vi "Calculate pO2-Rev3.vi"(10 "Spectral Data":T4={"PDT Amp [v]"=0.0, "RIS Amp [v]"=0.0, "B-Field"=[], "All In-Phase Scan Spectra"=[], "Model Select"=enum."OneCompRISTwoPDT", "Fit Each Scan"=FALSE, "PDT Center [g]"=0.0, "In-Phase Average Spectra"=[], "In-Phase Median Spectra"=[], "Out-Phase Median Spectra"=[], "Out-Phase Average Spectra"=[], "Fit Spectra"=[], "Fit No-Baseline Spectra"=[], "All Out-Phase Scan Spectra"=[], "Baseline Offset Correction"=FALSE, "In-Phase Offset [v]"=0.0, "Out-Phase Offset [v]"=0.0, "Ch2 Input\n(Balance)"=[], "Ch3 Input\n(Phase)"=[], "Ch4 Input\n(AFC)"=[], "Fit Pars"=[], "Fit Pars Errors"=[], "Fit Pars Labels"=[], "Raw Scan DAQ Data"=[], "Bad Scans Indicies"=[], "Good In-Phase Scan Spectra"=[], "Good Out-Phase Scan Spectra"=[], "Bad In-Phase Scan Spectra"=[], "Bad Out-Phase Scan Spectra"=[], "Number of bad scans"=0, "Fit History"=[], "PDT Amp. History/Set [v]"=[], "RIS Amp. History/Set [v]"=[], "RIS Amp. History/Scan [v]"=[], "All Shifted B-Fields"=[], "Good Shifted B-Fields"=[], "Ch5 Input\n(SpO2)"=[], "Ch6 Input\n(BPM)"=[], "Global SNR"=0.0, "Fit Error History"=[], "SNR History"=[]} {"Global SNR" min=0.0; "PDT Center [g]" min=0.0; "RIS Amp [v]" min=0.0; "PDT Amp [v]" min=0.0}, 11 "Measurement Information":T1={"Comments"="", "Directory Input"="", "Data file path"=path "C:/Data/EPR Data", "Scripting File"=path "C:/Data/Configuration Script.csv", "Save Data"=FALSE, "Tooth size (d11) [mm]"=0.0, "Tooth size (d12) [mm]"=0.0, "Tooth size (d21) [mm]"=0.0, "Tooth size (d22) [mm]"=0.0, "Dose of Tooth [Gy]"=0.0, "Safe Shutdown?"=FALSE, "Gases Available"=[], "Database Username"="", "Database Password"="", "Database Login URL"="", "Database Upload URL"="", "Database Success URL"="", "Database XML URL"="", "Database Resonator URL"="", "Session Number"=0, "Set #"=0, "Resonator Operator"="", "Session Type"="", "Tooth/Sample ID"="", "Volunteer ID"="", "Computer Operator"="", "Volunteer Type"="", "Site/Tooth Selection (T8,T9)"="", "Resonator"="", "Measurement Site"="", "Non-standard session?"=FALSE, "EPR DAQ Version"="", "Session Path"=path "C:/Data/EPR Data", "Chosen Applied State"="", "Chosen Initial State"="", "Time of Transition"="", "DAQ Mode"=enum."Engineering", "pO2/Scan [mmHg]"=[], "pO2/Set [mmHg]"=[], "Linewidth (HWHM)/Scan [Gauss]"=[], "Linewidth (HWHM)/Set [Gauss]"=[], "pO2 Conversion"="", "Dose Calibration Cluster"={"Dose Response"={"grand_mean"=0.0292016, "slope"=0.0188720543}, "Dose Correction"={"Sex"=1, "a0"=7.719669421, "a1"=-2.746550736, "a2"=-0.186490355, "a3"=0.041922063, "a4"=-0.849147359, "a5"=0.14330063, "a6"=0.019930219, "A_n"=40.0, "H_n"=10.12, "Dose Correction"=FALSE}, "Dose Reporting"={"Reporting is"=TRUE, "sd_threshold [AU]"=0.06, "sd_model [Gy]"=0.66, "dosimetric_threshold [Gy]"=2.0, "Add intrasession errors is"=FALSE, "Prior Radiation?"=FALSE}}, "OxyChip Slope"=0.0, "OxyChip Intercept"=0.0, "QA Mode"=enum."Select QA Mode", "QA Session?"=FALSE, "Sample Type"=enum."Empty Resonator", "Report pO2/Scan"=FALSE, "Skip End Session Save"=FALSE, "Number of sites"=enum."# Probes", "Recipient Name"="", "Sender Name"="", "Recipient Email"="", "Transition State History"=[], "pO2 Report Times"=[], "Temperature [C]"=0.0, "+Error pO2/Scan [mmHg]"=[], "-Error pO2/Scan [mmHg]"=[], "+Error pO2/Set [mmHg]"=[], "-Error pO2/Set [mmHg]"=[], "Oxy Phase Exclusion Tolerance [rad]"=0.0, "Oxy Center Exclusion Tolerance [%]"=0.0, "Oxy Exclude Unacceptable"=FALSE, "Oxy Unacceptable Estimate Flags"=[], "Save Session PPT"=FALSE, "Flagged Bad Sets"=[]} {"Oxy Center Exclusion Tolerance [%]" format="%#_9g"; "Oxy Phase Exclusion Tolerance [rad]" format="%#_9g"; "Temperature [C]" format="%#_9g"; "OxyChip Intercept" format="%#_9g"; "OxyChip Slope" format="%#_9g"; "Dose Calibration Cluster"."Dose Reporting"."dosimetric_threshold [Gy]" format="%#_9g"; "Dose Calibration Cluster"."Dose Reporting"."sd_model [Gy]" format="%#_9g"; "Dose Calibration Cluster"."Dose Reporting"."sd_threshold [AU]" format="%#_9g"; "Dose Calibration Cluster"."Dose Correction"."H_n" format="%#_9g"; "Dose Calibration Cluster"."Dose Correction"."A_n" format="%#_9g"; "Dose Calibration Cluster"."Dose Correction"."a6" format="%#.9g"; "Dose Calibration Cluster"."Dose Correction"."a5" format="%#.9g"; "Dose Calibration Cluster"."Dose Correction"."a4" format="%#.9g"; "Dose Calibration Cluster"."Dose Correction"."a3" format="%#.9g"; "Dose Calibration Cluster"."Dose Correction"."a2" format="%#.9g"; "Dose Calibration Cluster"."Dose Correction"."a1" format="%#.9g"; "Dose Calibration Cluster"."Dose Correction"."a0" format="%#.9g"; "Dose Calibration Cluster"."Dose Correction"."Sex" items=["Male"=1, "Female"=0]; "Dose Calibration Cluster"."Dose Response"."slope" format="%#_9g"; "Dose Calibration Cluster"."Dose Response"."grand_mean" format="%#_9g"}) -> (0 "pO2 Conversion":string, 1 "pO2 [mmHg]":dbl[](array[numeric]), 3 "Measurement Information Out":T1={"Comments"="", "Directory Input"="", "Data file path"=path "C:/Data/EPR Data", "Scripting File"=path "C:/Data/Configuration Script.csv", "Save Data"=FALSE, "Tooth size (d11) [mm]"=0.0, "Tooth size (d12) [mm]"=0.0, "Tooth size (d21) [mm]"=0.0, "Tooth size (d22) [mm]"=0.0, "Dose of Tooth [Gy]"=0.0, "Safe Shutdown?"=FALSE, "Gases Available"=[], "Database Username"="", "Database Password"="", "Database Login URL"="", "Database Upload URL"="", "Database Success URL"="", "Database XML URL"="", "Database Resonator URL"="", "Session Number"=0, "Set #"=0, "Resonator Operator"="", "Session Type"="", "Tooth/Sample ID"="", "Volunteer ID"="", "Computer Operator"="", "Volunteer Type"="", "Site/Tooth Selection (T8,T9)"="", "Resonator"="", "Measurement Site"="", "Non-standard session?"=FALSE, "EPR DAQ Version"="", "Session Path"=path "C:/Data/EPR Data", "Chosen Applied State"="", "Chosen Initial State"="", "Time of Transition"="", "DAQ Mode"=enum."Engineering", "pO2/Scan [mmHg]"=[], "pO2/Set [mmHg]"=[], "Linewidth (HWHM)/Scan [Gauss]"=[], "Linewidth (HWHM)/Set [Gauss]"=[], "pO2 Conversion"="", "Dose Calibration Cluster"={"Dose Response"={"grand_mean"=0.0292016, "slope"=0.0188720543}, "Dose Correction"={"Sex"=1, "a0"=7.719669421, "a1"=-2.746550736, "a2"=-0.186490355, "a3"=0.041922063, "a4"=-0.849147359, "a5"=0.14330063, "a6"=0.019930219, "A_n"=40.0, "H_n"=10.12, "Dose Correction"=FALSE}, "Dose Reporting"={"Reporting is"=TRUE, "sd_threshold [AU]"=0.06, "sd_model [Gy]"=0.66, "dosimetric_threshold [Gy]"=2.0, "Add intrasession errors is"=FALSE, "Prior Radiation?"=FALSE}}, "OxyChip Slope"=0.0, "OxyChip Intercept"=0.0, "QA Mode"=enum."Select QA Mode", "QA Session?"=FALSE, "Sample Type"=enum."Empty Resonator", "Report pO2/Scan"=FALSE, "Skip End Session Save"=FALSE, "Number of sites"=enum."# Probes", "Recipient Name"="", "Sender Name"="", "Recipient Email"="", "Transition State History"=[], "pO2 Report Times"=[], "Temperature [C]"=0.0, "+Error pO2/Scan [mmHg]"=[], "-Error pO2/Scan [mmHg]"=[], "+Error pO2/Set [mmHg]"=[], "-Error pO2/Set [mmHg]"=[], "Oxy Phase Exclusion Tolerance [rad]"=0.0, "Oxy Center Exclusion Tolerance [%]"=0.0, "Oxy Exclude Unacceptable"=FALSE, "Oxy Unacceptable Estimate Flags"=[], "Save Session PPT"=FALSE, "Flagged Bad Sets"=[]} {"Oxy Center Exclusion Tolerance [%]" format="%#_9g"; "Oxy Phase Exclusion Tolerance [rad]" format="%#_9g"; "Temperature [C]" format="%#_9g"; "OxyChip Intercept" format="%#_9g"; "OxyChip Slope" format="%#_9g"; "Dose Calibration Cluster"."Dose Reporting"."dosimetric_threshold [Gy]" format="%#_9g"; "Dose Calibration Cluster"."Dose Reporting"."sd_model [Gy]" format="%#_9g"; "Dose Calibration Cluster"."Dose Reporting"."sd_threshold [AU]" format="%#_9g"; "Dose Calibration Cluster"."Dose Correction"."H_n" format="%#_9g"; "Dose Calibration Cluster"."Dose Correction"."A_n" format="%#_9g"; "Dose Calibration Cluster"."Dose Correction"."a6" format="%#.9g"; "Dose Calibration Cluster"."Dose Correction"."a5" format="%#.9g"; "Dose Calibration Cluster"."Dose Correction"."a4" format="%#.9g"; "Dose Calibration Cluster"."Dose Correction"."a3" format="%#.9g"; "Dose Calibration Cluster"."Dose Correction"."a2" format="%#.9g"; "Dose Calibration Cluster"."Dose Correction"."a1" format="%#.9g"; "Dose Calibration Cluster"."Dose Correction"."a0" format="%#.9g"; "Dose Calibration Cluster"."Dose Correction"."Sex" items=["Male"=1, "Female"=0]; "Dose Calibration Cluster"."Dose Response"."slope" format="%#_9g"; "Dose Calibration Cluster"."Dose Response"."grand_mean" format="%#_9g"}, 4 "Negative pO2 Error [mmHg]":dbl[](array[numeric]), 6 "Positive pO2 Error [mmHg]":dbl[](array[numeric]))   [LabVIEW 2016]
uses:
  Types/Measurement Information.ctl
  Dose Calculation and Reporting/Dose Calculation Control.ctl
  Types/Sample Type.ctl
  Types/Spectral Data.ctl
  Types/Fitting Model Selection.ctl
panel:
  # "Session Information"
  # "Oximetric Data and Information"
  # "Email"
  # "Tooth Information"
  # "Database"
  # "Session Information"
  # "Oximetric Data and Information"
  # "Email"
  # "Tooth Information"
  # "Database"
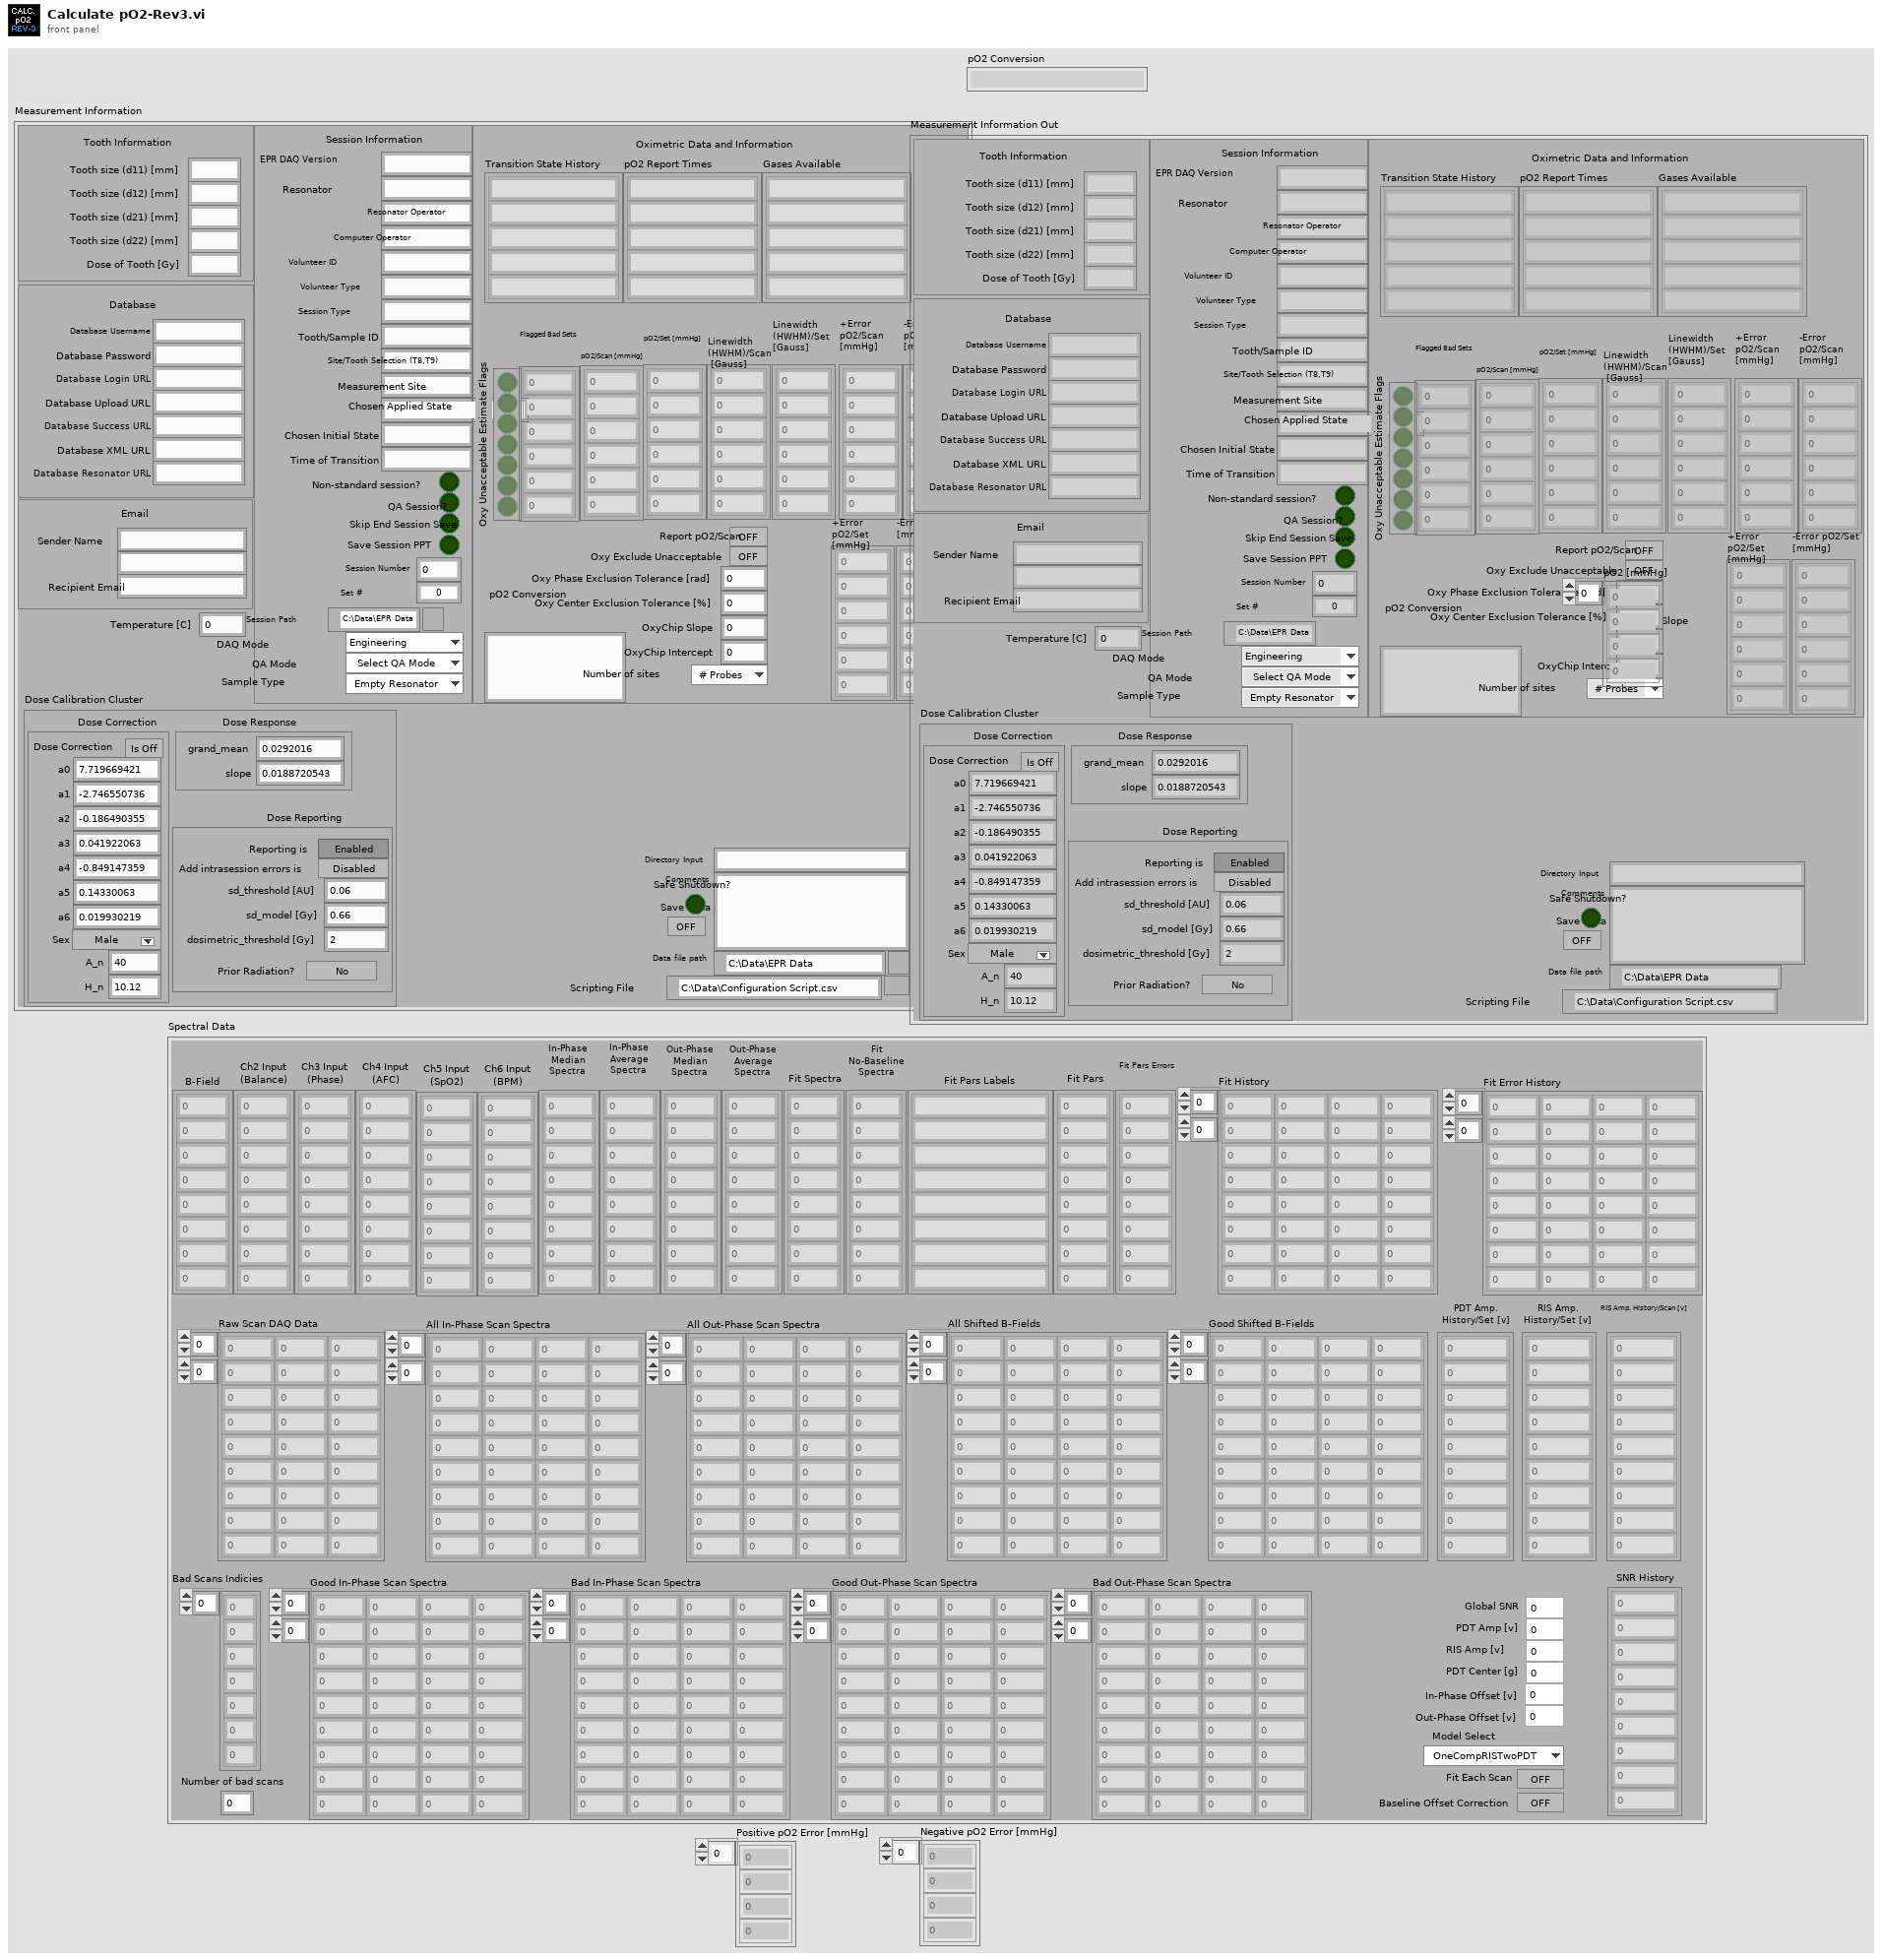
[diagram p1: front panel]
types:
  T1 = typedef "Measurement Information.ctl" = cluster{"Comments":string, "Directory Input":string, "Data file path":path, "Scripting File":path, "Save Data":bool, "Tooth size (d11) [mm]":dbl, "Tooth size (d12) [mm]":dbl, "Tooth size (d21) [mm]":dbl, "Tooth size (d22) [mm]":dbl, "Dose of Tooth [Gy]":dbl, "Safe Shutdown?":bool, "Gases Available":string[], "Database Username":string, "Database Password":string, "Database Login URL":string, "Database Upload URL":string, "Database Success URL":string, "Database XML URL":string, "Database Resonator URL":string, "Session Number":i32, "Set #":u32, "Resonator Operator":string, "Session Type":string, "Tooth/Sample ID":string, "Volunteer ID":string, "Computer Operator":string, "Volunteer Type":string, "Site/Tooth Selection (T8,T9)":string, "Resonator":string, "Measurement Site":string, "Non-standard session?":bool, "EPR DAQ Version":string, "Session Path":path, "Chosen Applied State":string, "Chosen Initial State":string, "Time of Transition":string, "DAQ Mode":enum16{"Engineering", "Dosimetry", "Oximetry"}, "pO2/Scan [mmHg]":dbl[][], "pO2/Set [mmHg]":dbl[][], "Linewidth (HWHM)/Scan [Gauss]":dbl[][], "Linewidth (HWHM)/Set [Gauss]":dbl[][], "pO2 Conversion":string, "Dose Calibration Cluster":T2, "OxyChip Slope":dbl, "OxyChip Intercept":dbl, "QA Mode":enum16{"Select QA Mode", "QA-Start/End", "QA-Mid", "QA-Weekly", "QA-Eng", "Check Calibration"}, "QA Session?":bool, "Sample Type":T3, "Report pO2/Scan":bool, "Skip End Session Save":bool, "Number of sites":enum16{"# Probes", "1", "2", "3", "4"}, "Recipient Name":string, "Sender Name":string, "Recipient Email":string, "Transition State History":string[], "pO2 Report Times":string[], "Temperature [C]":dbl, "+Error pO2/Scan [mmHg]":dbl[][], "-Error pO2/Scan [mmHg]":dbl[][], "+Error pO2/Set [mmHg]":dbl[][], "-Error pO2/Set [mmHg]":dbl[][], "Oxy Phase Exclusion Tolerance [rad]":dbl, "Oxy Center Exclusion Tolerance [%]":dbl, "Oxy Exclude Unacceptable":bool, "Oxy Unacceptable Estimate Flags":bool[], "Save Session PPT":bool, "Flagged Bad Sets":u32[]}
  T2 = typedef "Dose Calculation Control.ctl" = cluster{"Dose Response":cluster{"grand_mean":dbl, "slope":dbl}, "Dose Correction":cluster{"Sex":u16, "a0":dbl, "a1":dbl, "a2":dbl, "a3":dbl, "a4":dbl, "a5":dbl, "a6":dbl, "A_n":dbl, "H_n":dbl, "Dose Correction":bool}, "Dose Reporting":cluster{"Reporting is":bool, "sd_threshold [AU]":dbl, "sd_model [Gy]":dbl, "dosimetric_threshold [Gy]":dbl, "Add intrasession errors is":bool, "Prior Radiation?":bool}}
  T3 = typedef "Sample Type.ctl" = enum16{"Empty Resonator", "IRS", "BallZero", "Irradiated Tooth", "Non-irradiated Tooth", "OxyChip", "LiPc", "PDT", "India Ink"}
  T4 = typedef "Spectral Data.ctl" = cluster{"PDT Amp [v]":dbl, "RIS Amp [v]":dbl, "B-Field":dbl[], "All In-Phase Scan Spectra":dbl[][], "Model Select":T5, "Fit Each Scan":bool, "PDT Center [g]":dbl, "In-Phase Average Spectra":dbl[], "In-Phase Median Spectra":dbl[], "Out-Phase Median Spectra":dbl[], "Out-Phase Average Spectra":dbl[], "Fit Spectra":dbl[], "Fit No-Baseline Spectra":dbl[], "All Out-Phase Scan Spectra":dbl[][], "Baseline Offset Correction":bool, "In-Phase Offset [v]":dbl, "Out-Phase Offset [v]":dbl, "Ch2 Input\n(Balance)":dbl[], "Ch3 Input\n(Phase)":dbl[], "Ch4 Input\n(AFC)":dbl[], "Fit Pars":dbl[], "Fit Pars Errors":dbl[], "Fit Pars Labels":string[], "Raw Scan DAQ Data":dbl[][], "Bad Scans Indicies":i32[], "Good In-Phase Scan Spectra":dbl[][], "Good Out-Phase Scan Spectra":dbl[][], "Bad In-Phase Scan Spectra":dbl[][], "Bad Out-Phase Scan Spectra":dbl[][], "Number of bad scans":i32, "Fit History":dbl[][], "PDT Amp. History/Set [v]":dbl[], "RIS Amp. History/Set [v]":dbl[], "RIS Amp. History/Scan [v]":dbl[], "All Shifted B-Fields":dbl[][], "Good Shifted B-Fields":dbl[][], "Ch5 Input\n(SpO2)":dbl[], "Ch6 Input\n(BPM)":dbl[], "Global SNR":dbl, "Fit Error History":dbl[][], "SNR History":dbl[]}
  T5 = typedef "Fitting Model Selection.ctl" = enum16{"OneCompRIS", "OneCompRISTwoPDT", "OneCompRISRev", "OneCompRISTwoPDTRev", "LiPc", "TwoLiPc", "ThreeLiPc", "FourLiPc", "PDTCalibration", "CE_Ink", "Printex", "MelaninTwoPDT"}
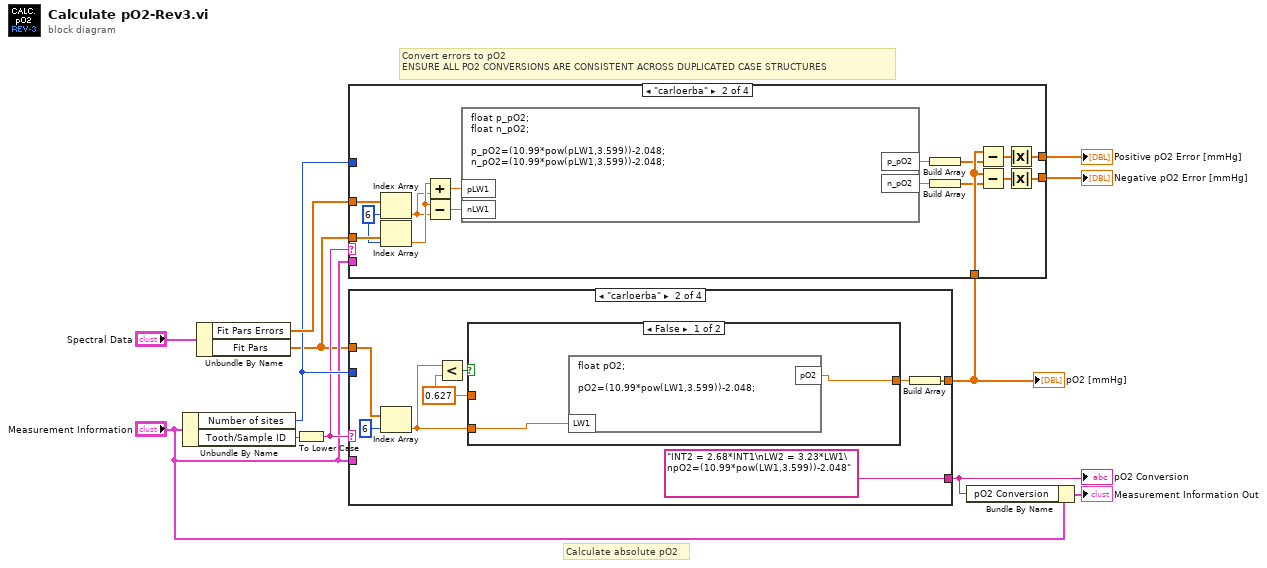
[diagram p0: block diagram]
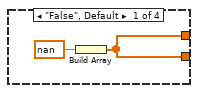
[diagram p2: hidden frame]
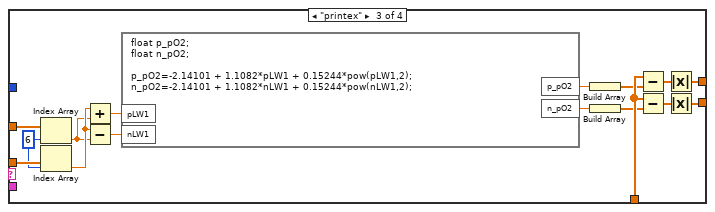
[diagram p3: hidden frame]
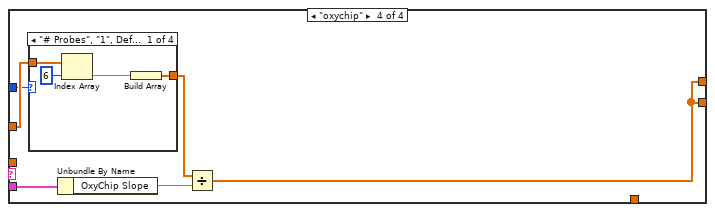
[diagram p4: hidden frame]
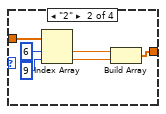
[diagram p5: hidden frame]
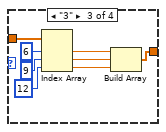
[diagram p6: hidden frame]
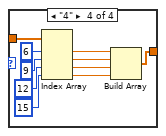
[diagram p7: hidden frame]
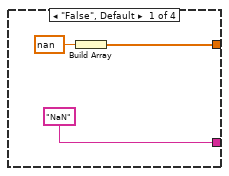
[diagram p8: hidden frame]
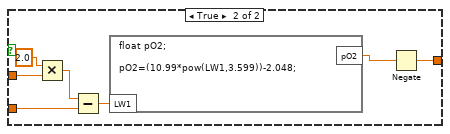
[diagram p9: hidden frame]
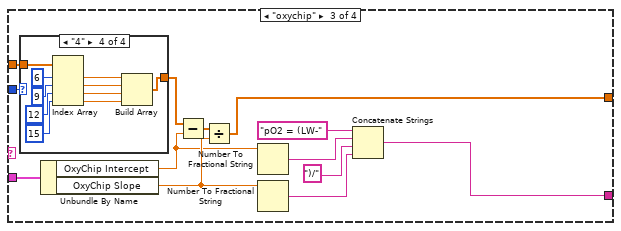
[diagram p10: hidden frame]
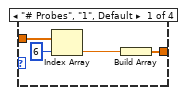
[diagram p11: hidden frame]
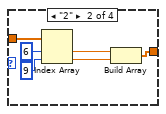
[diagram p12: hidden frame]
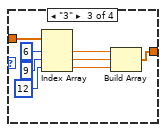
[diagram p13: hidden frame]
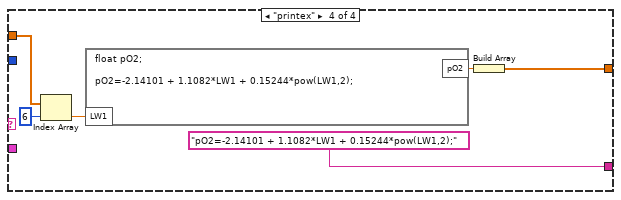
[diagram p14: hidden frame]
diagram:
  # "Calculate absolute pO2"
  # "Convert errors to pO2\nENSURE ALL PO2 CONVERSIONS ARE CONSISTENT ACROSS DUPLICATED CASE STRUCTURES"
  n1 = Unbundle By Name("Measurement Information") -> ("Number of sites"=w7:enum16{"# Probes", "1", "2", "3", "4"}, "Tooth/Sample ID"=w12:string)
  n2 = Unbundle By Name("Spectral Data") -> ("Fit Pars Errors"=w8:dbl[], "Fit Pars"=w4:dbl[])
  n3 = To Lower Case(string=w12) -> (all lower case string=w6:string)
  n4 = case shown="\"carloerba\"" w6 {
    tunnel: [w13 w20 w43 w74] -> w3
    tunnel: w4 -> [_ w22 w39 w76]
    tunnel: ["NaN" ("all lower case string") "INT2 = 2.68*INT1\nLW2 = 3.23*LW1\npO2=(10.99*pow(LW1,3.599))-2.048" ("all lower case string") w40 "pO2=-2.14101 + 1.1082*LW1 + 0.15244*pow(LW1,2);" ("all lower case string")] -> w10
    tunnel: "Measurement Information" -> [_ _ w45 _]
    tunnel: w7 -> [_ _ w37 _]
    frame "False", Default {
      n5 = Build Array(nan) -> (w13:dbl[])
    }
    frame "carloerba" {
      w16 = 0.627 ("y")
      n6 = Index Array(array=w22, index=6) -> (element=w17:dbl)
      n7 = Less?(x=w17, y=w16) -> (x < y?=w18:bool)
      n8 = case shown="False" w18 {
        tunnel: w17 -> [w25 w29]
        tunnel: [w24 w26] -> w19
        tunnel: w16 -> [_ w32]
        frame False {
          n9 = formula code="float pO2;\n\npO2=(10.99*pow(LW1,3.599))-2.048;"("LW1"=w25) -> ("pO2"=w24:dbl)
        }
        frame True {
          n10 = Multiply(x=2.0, y=w32) -> (x*y=w30:dbl)
          n11 = Subtract(x=w30, y=w29) -> (x-y=w28:dbl)
          n12 = formula code="float pO2;\n\npO2=(10.99*pow(LW1,3.599))-2.048;"("LW1"=w28) -> ("pO2"=w27:dbl)
          n13 = Negate(x=w27) -> (-x=w26:dbl)
        }
      }
      n14 = Build Array(w19) -> (w20:dbl[])
    }
    frame "oxychip" {
      n15 = case shown="\"4\"" w37 {
        tunnel: [w48 w54 w62 w72] -> w38
        tunnel: w39 -> [w46 w52 w60 w70]
        frame "# Probes", "1", Default {
          n16 = Index Array(array=w46, index=6) -> (element=w47:dbl)
          n17 = Build Array(w47) -> (w48:dbl[])
        }
        frame "2" {
          n18 = Index Array(array=w52, index #1=6 ("index"), index #2=9 ("index")) -> (element #1=w53:dbl, element #2=w50:dbl)
          n19 = Build Array(w53, w50) -> (w54:dbl[])
        }
        frame "3" {
          n20 = Index Array(array=w60, index #1=6 ("index"), index #2=9 ("index"), index #3=12 ("index")) -> (element #1=w61:dbl, element #2=w58:dbl, element #3=w56:dbl)
          n21 = Build Array(w61, w58, w56) -> (w62:dbl[])
        }
        frame "4" {
          n22 = Index Array(array=w70, index #1=6 ("index"), index #2=9 ("index"), index #3=12 ("index"), index #4=15 ("index")) -> (element #1=w71:dbl, element #2=w68:dbl, element #3=w66:dbl, element #4=w64:dbl)
          n23 = Build Array(w71, w68, w66, w64) -> (w72:dbl[])
        }
      }
      n24 = Unbundle By Name(w45) -> ("OxyChip Intercept"=w35:dbl, "OxyChip Slope"=w36:dbl)
      n25 = Subtract(x=w38, y=w35) -> (x-y=w44:dbl[])
      n26 = Divide(x=w44, y=w36) -> (x/y=w43:dbl[])
      n27 = Number To Fractional String(number=w35) -> (F-format string=w34:string)  [unwired: 3 in]
      n28 = Number To Fractional String(number=w36) -> (F-format string=w33:string)  [unwired: 3 in]
      n29 = Concatenate Strings("pO2 = (LW-" ("string"), w34, ")/" ("string"), w33) -> (w40:string)
    }
    frame "printex" {
      n30 = Index Array(array=w76, index=6) -> (element=w78:dbl)
      n31 = formula code="float pO2;\n\npO2=-2.14101 + 1.1082*LW1 + 0.15244*pow(LW1,2);"("LW1"=w78) -> ("pO2"=w77:dbl)
      n32 = Build Array(w77) -> (w74:dbl[])
    }
  }
  "pO2 Conversion" <- w10
  "pO2 [mmHg]" <- w3
  n33 = case shown="\"carloerba\"" w6 {
    tunnel: [w80 w82 w99 w114] -> w2
    tunnel: w8 -> [_ w97 w113 w118]
    tunnel: "Measurement Information" -> [_ _ _ w119]
    tunnel: w7 -> [_ _ _ w117]
    tunnel: [w80 w83 w98 w114] -> w1
    tunnel: w4 -> [_ w95 w111 _]
    tunnel: w3 -> [_ w86 w102 _]
    frame "False", Default {
      n34 = Build Array(nan) -> (w80:dbl[])
    }
    frame "carloerba" {
      w94 = 6 ("index")
      n35 = Index Array(array=w97, index=w94) -> (element=w89:dbl)
      n36 = Index Array(array=w95, index=w94) -> (element=w90:dbl)
      n37 = Add(x=w90, y=w89) -> (x+y=w93:dbl)
      n38 = Subtract(x=w90, y=w89) -> (x-y=w92:dbl)
      n39 = formula code="float p_pO2;\nfloat n_pO2;\n\np_pO2=(10.99*pow(pLW1,3.599))-2.048;\nn_pO2=(10.99*pow(pLW1,3.599))-2.048;"("pLW1"=w93, "nLW1"=w92) -> ("p_pO2"=w96:dbl, "n_pO2"=w91:dbl)
      n40 = Build Array(w96) -> (w85:dbl[])
      n41 = Build Array(w91) -> (w84:dbl[])
      n42 = Subtract(x=w86, y=w85) -> (x-y=w87:dbl[])
      n43 = Subtract(x=w86, y=w84) -> (x-y=w88:dbl[])
      n44 = Absolute Value(x=w87) -> (abs(x)=w82:dbl[])
      n45 = Absolute Value(x=w88) -> (abs(x)=w83:dbl[])
    }
    frame "printex" {
      w110 = 6 ("index")
      n46 = Index Array(array=w113, index=w110) -> (element=w105:dbl)
      n47 = Index Array(array=w111, index=w110) -> (element=w106:dbl)
      n48 = Add(x=w106, y=w105) -> (x+y=w109:dbl)
      n49 = Subtract(x=w106, y=w105) -> (x-y=w108:dbl)
      n50 = formula code="float p_pO2;\nfloat n_pO2;\n\np_pO2=-2.14101 + 1.1082*pLW1 + 0.15244*pow(pLW1,2);\nn_pO2=-2.14101 + 1.1082*nLW1 + 0.15244*pow(nLW1,2);"("pLW1"=w109, "nLW1"=w108) -> ("p_pO2"=w112:dbl, "n_pO2"=w107:dbl)
      n51 = Build Array(w112) -> (w100:dbl[])
      n52 = Build Array(w107) -> (w101:dbl[])
      n53 = Subtract(x=w102, y=w100) -> (x-y=w103:dbl[])
      n54 = Subtract(x=w102, y=w101) -> (x-y=w104:dbl[])
      n55 = Absolute Value(x=w103) -> (abs(x)=w99:dbl[])
      n56 = Absolute Value(x=w104) -> (abs(x)=w98:dbl[])
    }
    frame "oxychip" {
      n57 = case shown="\"# Probes\", \"1\", Default" w117 {
        tunnel: [w122 w128 w136 w146] -> w115
        tunnel: w118 -> [w120 w126 w134 w144]
        frame "# Probes", "1", Default {
          n58 = Index Array(array=w120, index=6) -> (element=w121:dbl)
          n59 = Build Array(w121) -> (w122:dbl[])
        }
        frame "2" {
          n60 = Index Array(array=w126, index #1=6 ("index"), index #2=9 ("index")) -> (element #1=w127:dbl, element #2=w124:dbl)
          n61 = Build Array(w127, w124) -> (w128:dbl[])
        }
        frame "3" {
          n62 = Index Array(array=w134, index #1=6 ("index"), index #2=9 ("index"), index #3=12 ("index")) -> (element #1=w135:dbl, element #2=w132:dbl, element #3=w130:dbl)
          n63 = Build Array(w135, w132, w130) -> (w136:dbl[])
        }
        frame "4" {
          n64 = Index Array(array=w144, index #1=6 ("index"), index #2=9 ("index"), index #3=12 ("index"), index #4=15 ("index")) -> (element #1=w145:dbl, element #2=w142:dbl, element #3=w140:dbl, element #4=w138:dbl)
          n65 = Build Array(w145, w142, w140, w138) -> (w146:dbl[])
        }
      }
      n66 = Unbundle By Name(w119) -> ("OxyChip Slope"=w116:dbl)
      n67 = Divide(x=w115, y=w116) -> (x/y=w114:dbl[])
    }
  }
  "Positive pO2 Error [mmHg]" <- w2
  "Negative pO2 Error [mmHg]" <- w1
  n68 = Bundle By Name(cluster="Measurement Information", "pO2 Conversion"=w10) -> (→"Measurement Information Out":T1)
